vi "validate mod cfg.vi"() -> ()   [LabVIEW 2013, in "TBM Tests.lvlib"]
uses:
  TBM Tests.lvlib
  module configuration/TBM module configuration.lvclass
panel:
  out "warn 538305":errorcluster
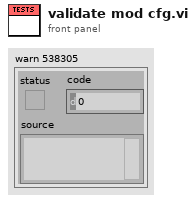
[diagram p1: front panel]
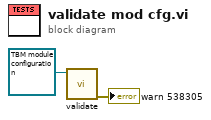
[diagram p0: block diagram]
diagram:
  n1 = call-dynamic "validate.vi"("configuration in"=refnum<class "TBM module configuration.lvclass"> refnum ("module configuration")) -> ("error out"=→"warn 538305":errorcluster)  [unwired: 9 in, 1 out]
